vi "HM8118 - Initialize.vi"(7 "Serial Configuration":T1={"Baud Rate"=9600, "Parity"=0, "Data Bits"=7, "Stop Bits"=10, "Flow Control"=0} {"Flow Control" items=["None", "XON/XOFF", "RTS/CTS", "XON/XOFF & RTS/CTS", "DTR/DSR", "XON/XOFF & DTR/DSR"]; "Stop Bits" items=["1.0"=10, "1.5"=15, "2.0"=20]; "Data Bits" items=["7"=7, "8"=8]; "Parity" items=["None", "Odd", "Even", "Mark", "Space"]; "Baud Rate" items=["300"=300, "600"=600, "1200"=1200, "2400"=2400, "4800"=4800, "9600"=9600, "19200"=19200]}, 8 "error in (no error)":errorcluster, 9 "Reset (True)":bool=TRUE, 10 "ID Query (True)":bool=TRUE, 11 "VISA resource name":refnum<visa-resource-name>) -> (0 "error out":errorcluster, 3 "VISA resource name out":refnum<visa-resource-name>)   [LabVIEW 2017]
doc: "Establishes communication with the instrument and optionally performs an instrument identification query and/or an instrument reset. It also places the instrument in a default state needed for other instrument driver operations. Therefore, call this VI before calling other instrument driver VIs for this instrument. Generally, you need to call the Initialize VI only once at the beginning of an application."
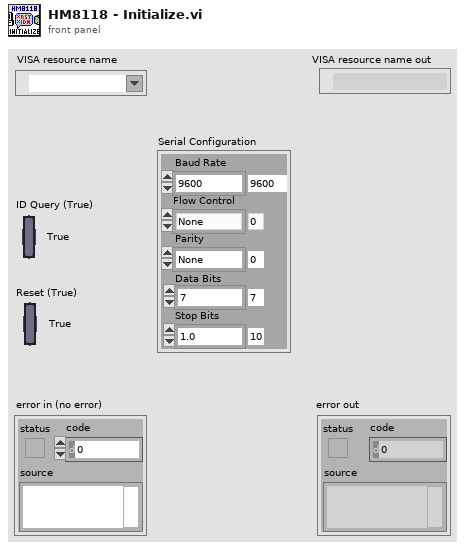
[diagram p1: front panel]
types:
  T1 = cluster{"Baud Rate":u32, "Parity":u16, "Data Bits":u16, "Stop Bits":u16, "Flow Control":u16}
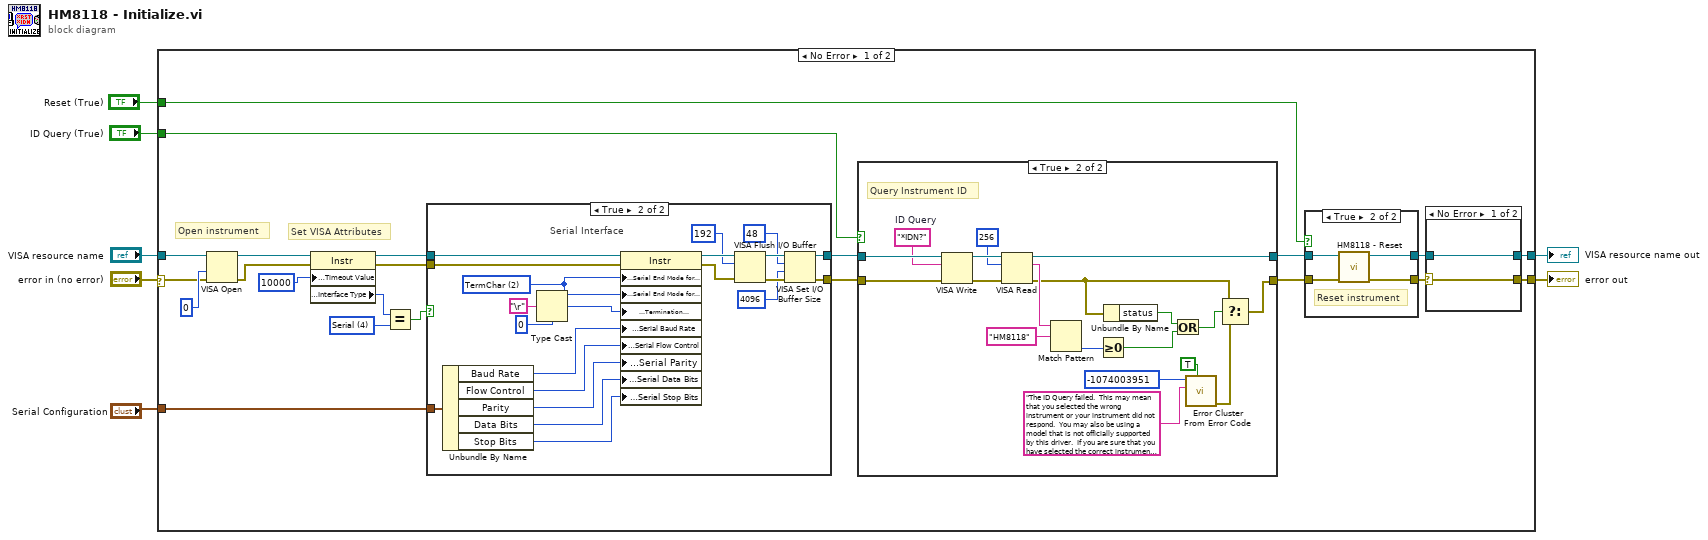
[diagram p0: block diagram]
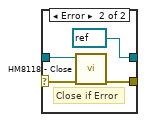
[diagram p3: hidden frame]
diagram:
  n1 = case shown="No Error" "error in (no error)" {
    selector: "error in (no error)" -> [w8 w87]
    tunnel: "ID Query (True)" -> [w27 _]
    tunnel: "Reset (True)" -> [w26 _]
    tunnel: "VISA resource name" -> [w25 w86]
    tunnel: [w15 w86] -> w4
    tunnel: [w14 w87] -> w3
    tunnel: "Serial Configuration" -> [w9 _]
    frame No Error {
      w17 = u16 4 items=["GPIB"=1, "VXI"=2, "GPIB-VXI"=3, "Serial"=4, "PXI"=5, "TCPIP"=6, "USB"=7] ("Interface Information:Interface Type")
      # "Set VISA Attributes"
      # "Open instrument"
      n2 = VISA Open(access mode=u32 0, error in (no error)=w8, VISA resource name=w25) -> (VISA resource name=w10:refnum<visa-resource-name>, error out=w11:errorcluster)  [unwired: 2 out]
      n3 = property on="Property Node" class="Instr"(reference=w10, error in=w11, "General Settings:Timeout Value"=u32 10000) -> (reference out=w20:refnum<visa-resource-name>, error out=w19:errorcluster, "Interface Information:Interface Type"=w24:u16)
      n4 = Equal?(x=w24, y=w17) -> (x = y?=w18:bool)
      n5 = case shown="True" w18 {
        tunnel: [w30 w49] -> w22
        tunnel: [w31 w46] -> w21
        tunnel: w20 -> [w30 w51]
        tunnel: w19 -> [w31 w52]
        tunnel: w9 -> [_ w32]
        frame False {
          # "GPIB Interface"
        }
        frame True {
          w39 = u16 2 items=["None", "LastBit", "TermChar"] ("Serial Settings:Serial End Mode for Reads")
          # "Serial Interface"
          n6 = Unbundle By Name(w32) -> ("Baud Rate"=w37:u32, "Flow Control"=w34:u16, "Parity"=w35:u16, "Data Bits"=w36:u16, "Stop Bits"=w33:u16)
          n7 = Type Cast(type=u8 0, x="\r") -> (*(type *) &x=w38:u8)
          n8 = property on="Property Node" class="Instr"(reference=w51, error in=w52, "Serial Settings:Serial End Mode for Reads"=w39, "Serial Settings:Serial End Mode for Writes"=w39, "Message Based Settings:Termination Character"=w38, "Serial Settings:Serial Baud Rate"=w37, "Serial Settings:Serial Flow Control"=w34, "Serial Settings:Serial Parity"=w35, "Serial Settings:Serial Data Bits"=w36, "Serial Settings:Serial Stop Bits"=w33) -> (reference out=w45:refnum<visa-resource-name>, error out=w48:errorcluster)
          n9 = VISA Flush I/O Buffer(VISA resource name=w45, mask (16)=u16 192, error in (no error)=w48) -> (VISA resource name out=w50:refnum<visa-resource-name>, error out=w47:errorcluster)
          n10 = VISA Set I/O Buffer Size(VISA resource name=w50, mask (16)=u16 48, size (4096)=u32 4096 ("size (0)"), error in (no error)=w47) -> (VISA resource name out=w49:refnum<visa-resource-name>, error out=w46:errorcluster)
        }
      }
      n11 = case shown="True" w27 {
        tunnel: [w65 w85] -> w28
        tunnel: [w66 w82] -> w29
        tunnel: w22 -> [w66 w83]
        tunnel: w21 -> [w65 w84]
        frame False {
        }
        frame True {
          w77 = "*IDN?"  # ID Query
          # "Query Instrument ID"
          n12 = VISA Write(VISA resource name=w83, write buffer=w77, error in (no error)=w84) -> (VISA resource name out=w80:refnum<visa-resource-name>, error out=w79:errorcluster)  [unwired: 1 out]
          n13 = VISA Read(VISA resource name=w80, byte count=u32 256, error in (no error)=w79) -> (VISA resource name out=w82:refnum<visa-resource-name>, read buffer=w81:string, error out=w71:errorcluster)  [unwired: 1 out]
          n14 = Match Pattern(string=w81, regular expression="HM8118") -> (offset past match=w72:i32)  [unwired: 4 out]
          n15 = Greater Or Equal To 0?(x=w72) -> (x >= 0?=w69:bool)
          n16 = Unbundle By Name(w71) -> ("status"=w70:bool)
          n17 = Or(x=w70, y=w69) -> (x .or. y?=w68:bool)
          n18 = call <vilib>:"Error Cluster From Error Code.vi"("show call chain? (False)"=TRUE, "error message (\"\")"="The ID Query failed.  This may mean that you selected the wrong instrument or your instrument did not respond.  You may also be using a model that is not officially supported by this driver.  If you are sure that you have selected the correct instrument and it is responding, try disabling the ID Query." ("Source (VI Name)"), "error code (0)"=-1074003951 ("Code")) -> ("error out"=w76:errorcluster)  [unwired: 1 in, 5 out]
          n19 = Select(t=w71, s=w68, f=w76) -> (s? t:f=w85:errorcluster)
        }
      }
      n20 = case shown="True" w26 {
        tunnel: w28 -> [w59 w62]
        tunnel: [w59 w61] -> w12
        tunnel: w29 -> [w60 w63]
        tunnel: [w60 w64] -> w13
        frame False {
        }
        frame True {
          # "Reset instrument"
          n21 = call "HM8118 - Reset.vi"("error in (no error)"=w62, "VISA resource name"=w63) -> ("error out"=w61:errorcluster, "VISA resource name out"=w64:refnum<visa-resource-name>)  [unwired: 8 in]
        }
      }
      n22 = case shown="No Error" w12 {
        selector: w12 -> [w53 w56]
        tunnel: w13 -> [w54 w57]
        tunnel: [w54 refnum<visa-resource-name> refnum ("VISA resource name out")] -> w15
        tunnel: [w53 w55] -> w14
        frame No Error {
        }
        frame Error {
          # "Close if Error"
          n23 = call "HM8118 - Close.vi"("VISA resource name"=w57, "error in (no error)"=w56) -> ("error out"=w55:errorcluster)  [unwired: 8 in]
        }
      }
    }
    frame Error {
    }
  }
  "VISA resource name out" <- w4
  "error out" <- w3
